vi "Config_CheckLS335.vi"(5 "Status Ref":refnum<vi>, 7 "HM 8119":refnum<vi>, 8 "error in (no error)":errorcluster, 10 "Config Cluster":T1={"General"={"Config.ini"=path "", "Default Logging Path"=path ""}, "Hardware"={"Measure Rate (1/s)"=0, "HP DMM VISA"="", "LS 335 VISA"="", "HP DM"={"Range"=enum."Autorange", "Autozero"=FALSE, "Display"=enum."3 1/2 Digit", "Blank LCD"=FALSE}, "LS335"={"Brightness"=enum."25%"}}, "Operation"={"Operation Mode"=enum."Idle-Off", "Status"="", "NewLog?"=FALSE, "OvenWarn"=FALSE, "LS335"={"Heater A"={"Range"=enum."Off", "Set Point"=0.0}, "Heater B"={"Range"=enum."Off", "Set Point"=0.0}}}}) -> (0 "error out":errorcluster, 1 "Connected?":bool, 2 "Config Cluster Out":T1={"General"={"Config.ini"=path "", "Default Logging Path"=path ""}, "Hardware"={"Measure Rate (1/s)"=0, "HP DMM VISA"="", "LS 335 VISA"="", "HP DM"={"Range"=enum."Autorange", "Autozero"=FALSE, "Display"=enum."3 1/2 Digit", "Blank LCD"=FALSE}, "LS335"={"Brightness"=enum."25%"}}, "Operation"={"Operation Mode"=enum."Idle-Off", "Status"="", "NewLog?"=FALSE, "OvenWarn"=FALSE, "LS335"={"Heater A"={"Range"=enum."Off", "Set Point"=0.0}, "Heater B"={"Range"=enum."Off", "Set Point"=0.0}}}})   [LabVIEW 2021]
uses:
  Config_Cluster.ctl
  Mode_Enum.ctl
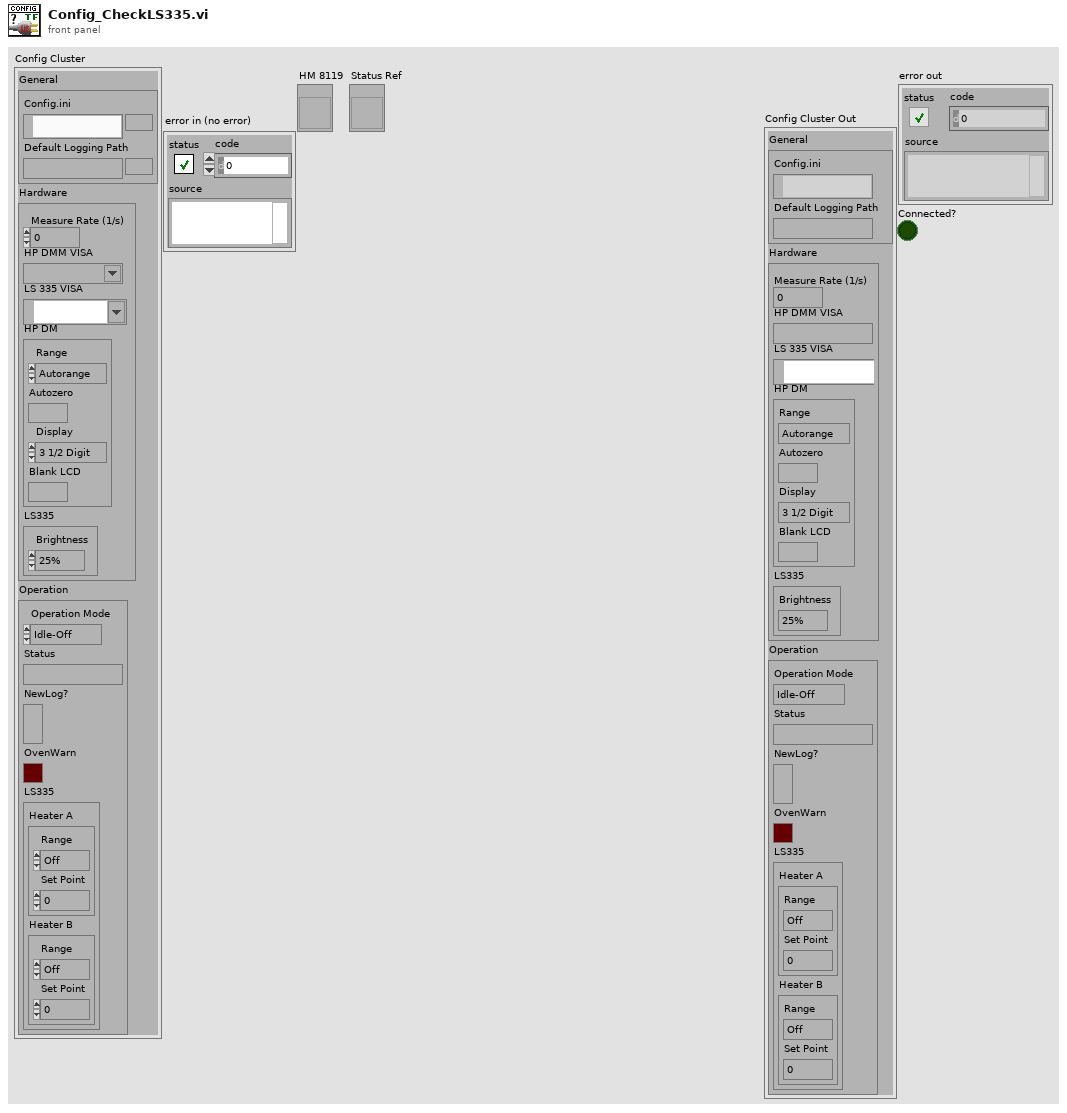
[diagram p1: front panel]
types:
  T1 = typedef "Config_Cluster.ctl" = cluster{"General":cluster{"Config.ini":path, "Default Logging Path":path}, "Hardware":cluster{"Measure Rate (1/s)":i32, "HP DMM VISA":refnum<visa-resource-name>, "LS 335 VISA":refnum<visa-resource-name>, "HP DM":cluster{"Range":enum16{"Autorange", "30mV", "300mV", "3V", "30V"}, "Autozero":bool, "Display":enum16{"3 1/2 Digit", "4 1/2 Digit", "5 1/2 Digit"}, "Blank LCD":bool}, "LS335":cluster{"Brightness":enum16{"25%", "50%", "75%", "100%"}}}, "Operation":cluster{"Operation Mode":T2, "Status":string, "NewLog?":bool, "OvenWarn":bool, "LS335":cluster{"Heater A":cluster{"Range":enum16{"Off", "Low", "Medium", "High"}, "Set Point":dbl}, "Heater B":cluster{"Range":enum16{"Off", "Low", "Medium", "High"}, "Set Point":dbl}}}}
  T2 = typedef "Mode_Enum.ctl" = enum16{"OvenNRDY", "Logging", "Idle-Off", "Idle"}
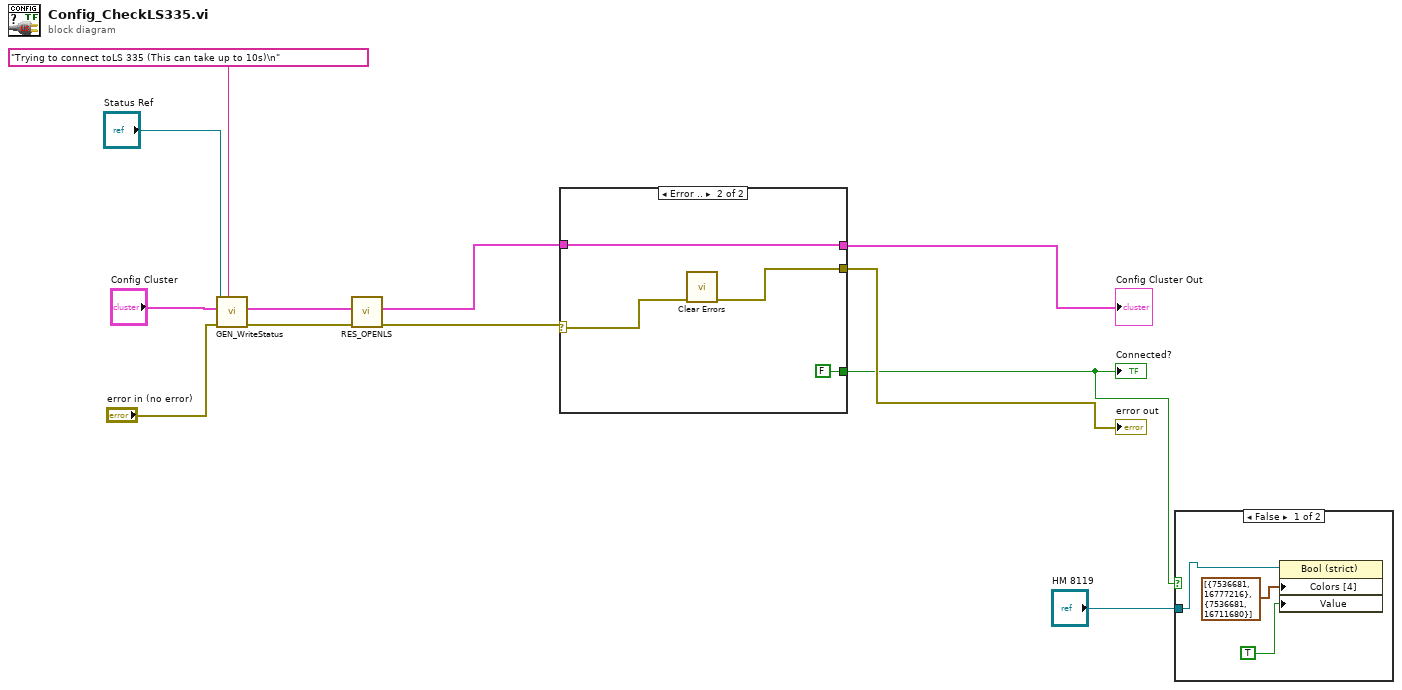
[diagram p0: block diagram]
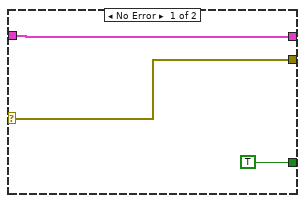
[diagram p2: hidden frame]
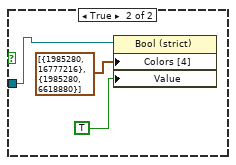
[diagram p3: hidden frame]
diagram:
  n1 = call "GEN_WriteStatus.vi"("Input String"="Trying to connect toLS 335 (This can take up to 10s)\n", "error in (no error)"="error in (no error)", "Config_Cluster"="Config Cluster", "Status Ref"="Status Ref") -> ("error out"=w1:errorcluster, "Config_Cluster Out"=w4:T1)  [unwired: 6 in]
  n2 = call "RES_OPENLS.vi"("error in (no error)"=w1, "Configuration Cluster"=w4) -> ("error out"=w2:errorcluster, "Configuration Cluster Out"=w3:T1)  [unwired: 8 in]
  n3 = case shown="Error .." w2 {
    selector: w2 -> [w14 w19]
    tunnel: w3 -> [w15 w16]
    tunnel: [w15 w16] -> w5
    tunnel: [w14 w18] -> w12
    tunnel: [TRUE FALSE] -> w11
    frame No Error {
    }
    frame Error {
      n4 = call <vilib>:"Clear Errors.vi"("error in (no error)"=w19) -> ("error out"=w18:errorcluster)  [unwired: 5 in, 1 out]
    }
  }
  "Config Cluster Out" <- w5
  "error out" <- w12
  "Connected?" <- w11
  n5 = case shown="False" w11 {
    tunnel: "HM 8119" -> [w20 w23]
    frame False {
      n6 = property class="Bool (strict)"(reference=w20, "Colors [4]"=cluster{u32, u32}[] [{7536681, 16777216}, {7536681, 16711680}], "Value"=TRUE) -> ()  [unwired: 1 in, 2 out]
    }
    frame True {
      n7 = property class="Bool (strict)"(reference=w23, "Colors [4]"=cluster{u32, u32}[] [{1985280, 16777216}, {1985280, 6618880}], "Value"=TRUE) -> ()  [unwired: 1 in, 2 out]
    }
  }
